vi "ProcessFileFlow_Name.vi"() -> (1 "message name":string)   [LabVIEW 2017, in "FileFlow.lvlib"]
uses:
  <vilib>/addons/InsightCM/Devices/Shared/Common/FileFlow/FileFlow.lvlib
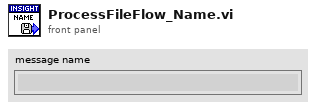
[diagram p1: front panel]
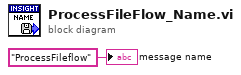
[diagram p0: block diagram]
diagram:
  "message name" <- "ProcessFileflow" ("ProcessName")
